vi "Scalar Bitpacked.vi"(8 "error in (no error)":errorcluster, 11 "Node Ptr":T1 format="%.0x") -> (0 "error out":errorcluster)   [LabVIEW 2018, in "FPGA Addon System Explorer.lvlib"]
uses:
  FPGA Addon System Explorer.lvlib
  <vilib>/NI VeriStand/Custom Device API/Custom Device API.lvlib
  Addon Shared/FPGA Addon Shared.lvlib
  Addon Shared/Types/FG Action.ctl
  Addon Shared/SubVIs/Constants.vi
  <vilib>/NI VeriStand/Custom Device API/Get Item Property (String).vi
  <vilib>/NI VeriStand/Custom Device API/Custom Device Item Ref.ctl
panel:
  out "Original Name":string
  in  "SHDocVw.IWebBrowser":refnum<k7>(container)
  in  "Reset":bool
  in  "Apply":bool
  in  "Number of Channels":u8
  in  "Header 2":cluster{"Section Name":string}={"Section Name"="Bitpacked Settings"}
  in  "Header":cluster{"Section Name":string}={"Section Name"="Section Settings"}
  in  "Description":string
  in  "Name":string
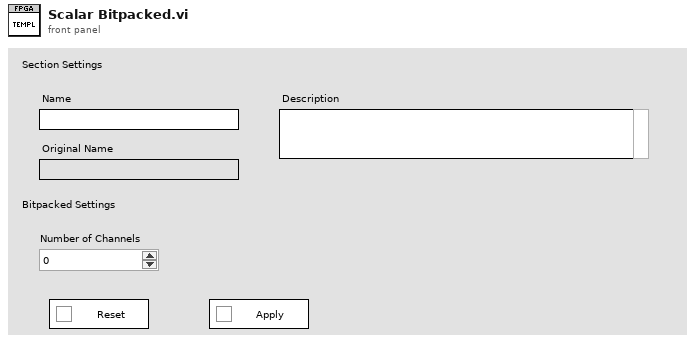
[diagram p1: front panel]
types:
  T1 = typedef "Custom Device API.lvlib/Custom Device Item Ref.ctl" = u64
  T2 = typedef "FPGA Addon Shared.lvlib/FG Action.ctl" = enum8{"GET", "SET"}
  T3 = typedef "FPGA Addon Shared.lvlib/Scalar Settings.ctl" = cluster{"Number of Channels":u8}
  T4 = typedef "FPGA Addon Shared.lvlib/Register Information.ctl" = cluster{"Name":string, "Data Type":T5, "Default Value":variant}
  T5 = typedef "FPGA Addon Shared.lvlib/Data Type.ctl" = enum8{"<Null>", "I8", "I16", "I32", "I64", "U8", "U16", "U32", "U64", "SGL", "Boolean", "Analog PWM In Settings", "Analog PWM In", "Digital PWM In Settings", "Digital PWM In", "Digital PWM Out", "Sine Out", "FXP+/-24.5", "FXP+/-16.5", "FXP+/-32.8", "FXP+/-64.32", "FXP+/-16.7", "FXP+/-20.5", "FXP+/-27.5", "FXP+/-32.16", "FXP+16.3", "FXP+18.3", "Digital Static In", "Digital Static Out", "Digital Static In Settings", "Digital WSS Out", "Quad Encoder Settings", "Quad Encoder In", "Group"}
  T6 = typedef "Custom Device API.lvlib/Custom Device Item Info.ctl" = cluster{"Name":string, "Is Channel":bool, "GUID":string, "Is Waveform":bool}
  T7 = typedef "Custom Device API.lvlib/Custom Device Commands.ctl" = enum16{"Default", "Item renamed", "Shutdown", "Dynamic button pressed"}
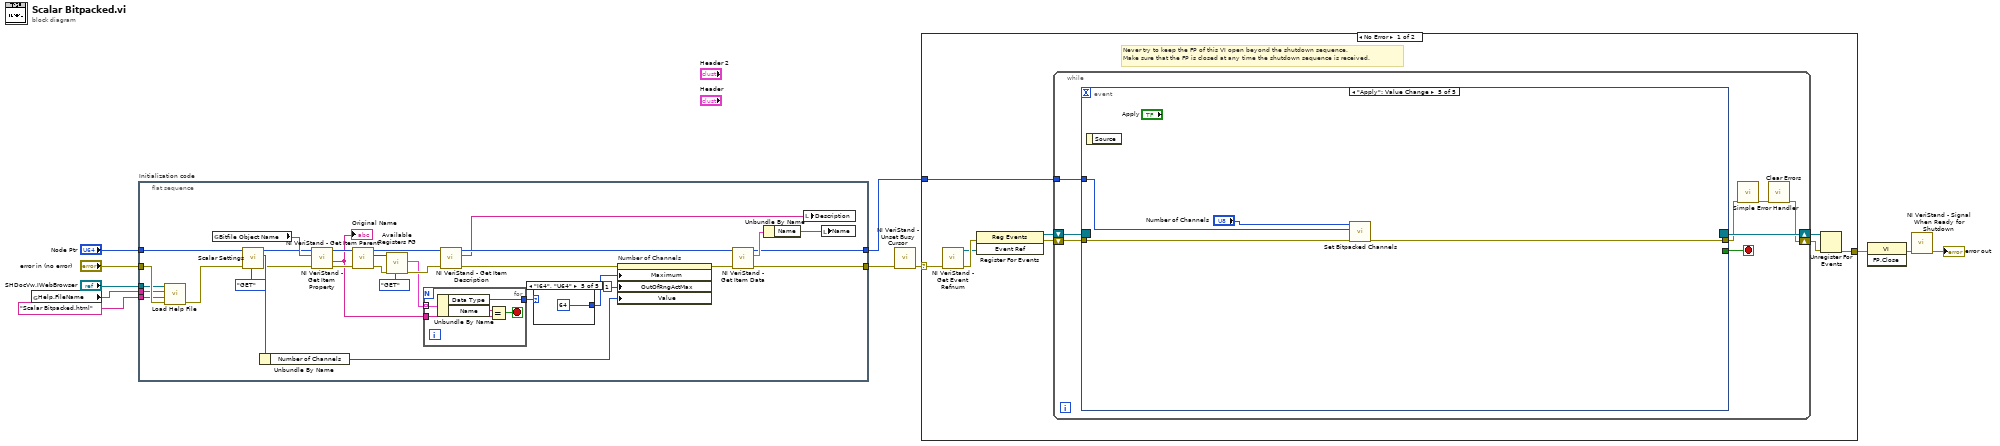
[diagram p0: block diagram]
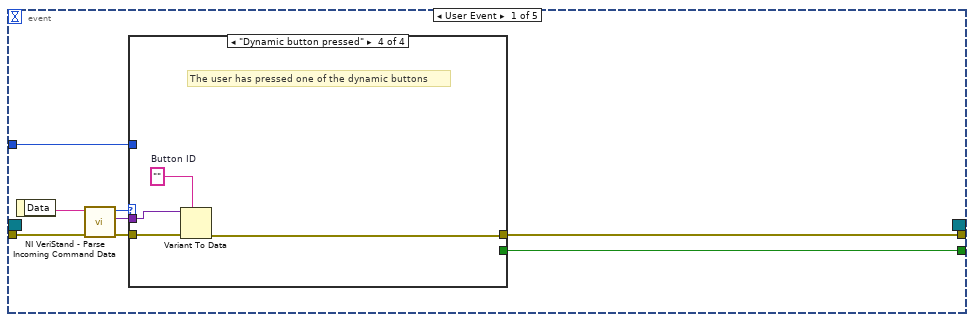
[diagram p2: hidden frame]
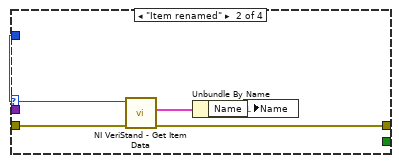
[diagram p4: hidden frame]
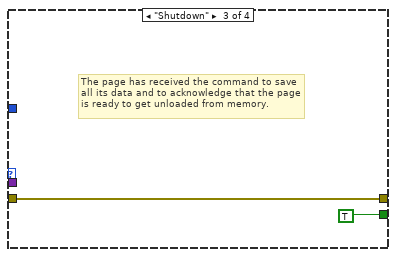
[diagram p5: hidden frame]
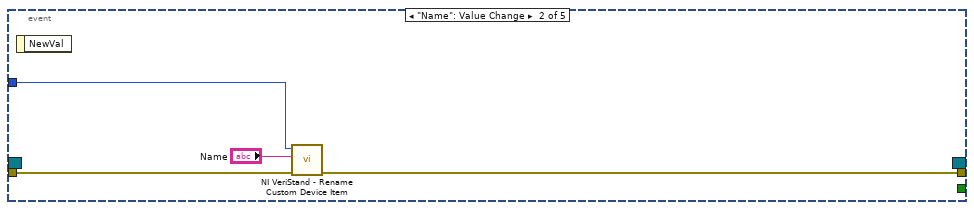
[diagram p6: hidden frame]
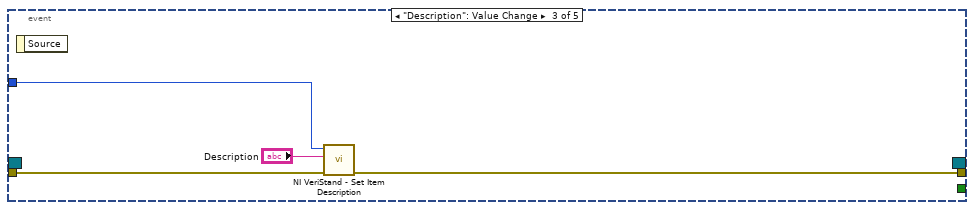
[diagram p7: hidden frame]
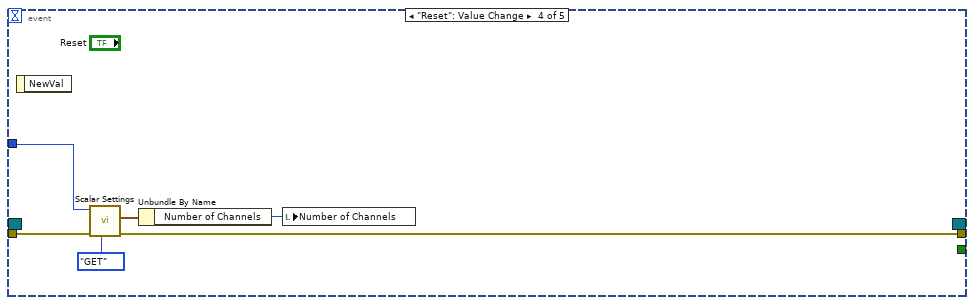
[diagram p8: hidden frame]
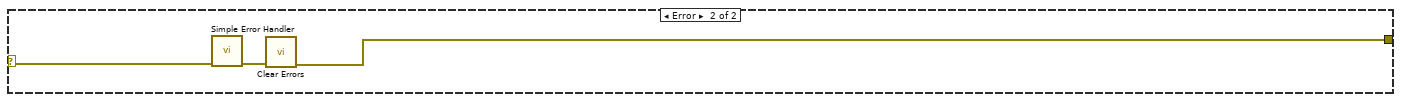
[diagram p9: hidden frame]
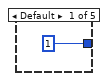
[diagram p10: hidden frame]
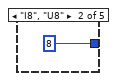
[diagram p11: hidden frame]
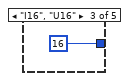
[diagram p12: hidden frame]
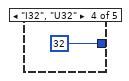
[diagram p13: hidden frame]
diagram:
  n1 = global read "Constants.vi" "Help.FileName"() -> (w1:string)
  n2 = flat-sequence "Initialization code" {
    tunnel: "error in (no error)" -> [w17]
    tunnel: "Node Ptr" -> [w25]
    tunnel: [w39] -> w8
    tunnel: [w40] -> w6
    tunnel: "SHDocVw.IWebBrowser" -> [w15]
    tunnel: w1 -> [w14]
    tunnel: "Scalar Bitpacked.html" ("HTML File") -> [w13]
    frame #0 {
      n3 = call "Load Help File.vi"("error in (no error)"=w17, "HTML File"=w13, "Main CHM File"=w14, "SHDocVw.IWebBrowser2"=w15) -> ("error out"=w16:errorcluster)  [unwired: 7 in]
      n4 = global read "Constants.vi" "Bitfile Object Name"() -> (w30:string)
      n5 = call "Scalar Settings.vi"("Action"=FG_Action."GET", "error in (no error)"=w16, "Item Ref"=w25) -> ("error out"=w24:errorcluster, "Scalar Settings"=w37:T3, "Item Ref out"=w23:T1)  [unwired: 6 in]
      n6 = Unbundle By Name(w37) -> ("Number of Channels"=w28:u8)
      n7 = call-poly <vilib>:"NI VeriStand - Get Item Property.vi"("error in (no error)"=w24, "Property Name"=w30, "Item Ref in"=w23) -> ("error out"=w21:errorcluster, "Value"=w12:string, "Item Ref out"=w22:T1)  [unwired: 5 in, 1 out]
      "Original Name" <- w12
      n8 = call <vilib>:"NI VeriStand - Get Item Parent.vi"("error in (no error)"=w21, "Item Ref in"=w22) -> ("error out"=w34:errorcluster, "Parent Ref"=w35:T1, "Item Ref out"=w36:T1)  [unwired: 6 in, 1 out]
      n9 = call "Available Registers FG.vi"("Action"=FG_Action."GET", "error in (no error)"=w34, "Item Ref"=w35) -> ("error out"=w33:errorcluster, "Available Registers"=w31:T4[])  [unwired: 6 in, 1 out]
      n10 = for {
        tunnel: w31 -> [w53] mode=indexing
        tunnel: w12 -> [w51]
        tunnel: [w49] -> w27
        stop <- w50 stop-if-true
        n11 = Unbundle By Name(w53) -> ("Data Type"=w49:T5, "Name"=w52:string)
        n12 = Equal?(x=w52, y=w51) -> (x = y?=w50:bool)
      }
      n13 = call <vilib>:"NI VeriStand - Get Item Description.vi"("error in (no error)"=w33, "Item Ref in"=w36) -> ("error out"=w20:errorcluster, "Description"=w42:string, "Item Ref out"=w43:T1)  [unwired: 7 out]
      n14 = case shown="\"I64\", \"U64\"" w27 {
        tunnel: [1 8 16 32 64] -> w26
        frame Default {
        }
        frame "I8", "U8" {
        }
        frame "I16", "U16" {
        }
        frame "I32", "U32" {
        }
        frame "I64", "U64" {
        }
      }
      n15 = property on="Number of Channels" class="DigNum (strict)"(error in=w20, "Maximum"=w26, "OutOfRngActMax"=u8 1 ("Response to Value Outside Limits:Maximum"), "Value"=w28) -> (error out=w19:errorcluster)  [unwired: 1 in, 1 out]
      n16 = call <vilib>:"NI VeriStand - Get Item Data.vi"("error in (no error)"=w19, "Item Ref in"=w43) -> ("error out"=w39:errorcluster, "Item Info"=w41:T6, "Item Ref out"=w40:T1)  [unwired: 7 out]
      n17 = Unbundle By Name(w41) -> ("Name"=w18:string)
      n18 = local write "Description"(w42) -> ()
      n19 = local write "Name"(w18) -> ()
    }
  }
  n20 = call <vilib>:"NI VeriStand - Unset Busy Cursor.vi"("error in (no error)"=w8) -> ("error out"=w7:errorcluster)  [unwired: 10 out]
  n21 = case shown="No Error" w7 {
    selector: w7 -> [w54 w111]
    tunnel: [w59 w109] -> w11
    tunnel: w6 -> [w55 _]
    frame No Error {
      # "Never try to keep the FP of this VI open beyond the shutdown sequence.\nMake sure that the FP is closed at any time the shutdown sequence is received."
      n22 = call <vilib>:"NI VeriStand - Get Event Refnum.vi"("error in (no error)"=w54) -> ("error out"=w62:errorcluster, "Event Ref"=w58:refnum<user-event>)  [unwired: 9 out]
      n23 = register-events(error in=w62, w58) -> (reference out=w56:refnum<event-registration>, error out=w57:errorcluster)  [unwired: 1 in]
      n24 = while {
        tunnel: w55 -> [w66]
        shift-right: [w63] -> w60
        shift-left: w57 -> [w69]
        shift-right: [w70] -> w61
        shift-left: w56 -> [w68]
        stop <- w67 stop-if-true
        n25 = event shown="[4] \"Apply\": Value Change" {
          selector: w68 -> [_ _ _ _ _]
          dyn-events: [_ _ _ _ _] -> w70
          timeout: _ -> [_ _ _ _ _]
          tunnel: w69 -> [w78 w94 w97 w104 w106]
          tunnel: [w74 _ _ _ _] -> w67
          tunnel: [w73 w93 w96 w100 w105] -> w65
          tunnel: w66 -> [w72 w92 w98 w102 w107]
          event User Event {
            n26 = event-data() -> ("Data"=w77:string)  [unwired: 1 out]
            n27 = call <vilib>:"NI VeriStand - Parse Incoming Command Data.vi"("error in (no error)"=w78, "Incoming data"=w77) -> ("error out"=w76:errorcluster, "Outgoing data"=w71:variant, "Action"=w75:T7)  [unwired: 7 out]
            n28 = case shown="\"Dynamic button pressed\"" w75 {
              tunnel: w76 -> [w79 w84 w85 w90]
              tunnel: [_ _ TRUE _] -> w74
              tunnel: [w79 w81 w85 w87] -> w73
              tunnel: w72 -> [_ w83 _ _]
              tunnel: w71 -> [_ _ _ w89]
              frame "Default", Default {
              }
              frame "Item renamed" {
                n29 = call <vilib>:"NI VeriStand - Get Item Data.vi"("error in (no error)"=w84, "Item Ref in"=w83) -> ("error out"=w81:errorcluster, "Item Info"=w82:T6)  [unwired: 8 out]
                n30 = Unbundle By Name(w82) -> ("Name"=w80:string)
                n31 = local write "Name"(w80) -> ()
              }
              frame "Shutdown" {
                # "The page has received the command to save all its data and to acknowledge that the page is ready to get unloaded from memory."
              }
              frame "Dynamic button pressed" {
                w88 = ""  # Button ID
                # "The user has pressed one of the dynamic buttons"
                n32 = Variant To Data(error in=w90, type=w88, Variant=w89) -> (error out=w87:errorcluster)  [unwired: 1 out]
              }
            }
          }
          event "Name": Value Change {
            n33 = event-data() -> ()  [unwired: 2 out]
            n34 = call <vilib>:"NI VeriStand - Rename Custom Device Item.vi"("error in (no error)"=w94, "New Name"="Name", "Item Ref in"=w92) -> ("error out"=w93:errorcluster)  [unwired: 1 in, 7 out]
          }
          event "Description": Value Change {
            n35 = event-data() -> ()  [unwired: 2 out]
            n36 = call <vilib>:"NI VeriStand - Set Item Description.vi"("error in (no error)"=w97, "Description"="Description", "Item Ref in"=w98) -> ("error out"=w96:errorcluster)  [unwired: 8 out]
          }
          event "Reset": Value Change {
            n37 = event-data() -> ()  [unwired: 2 out]
            n38 = call "Scalar Settings.vi"("Action"=FG_Action."GET", "error in (no error)"=w104, "Item Ref"=w102) -> ("error out"=w100:errorcluster, "Scalar Settings"=w101:T3)  [unwired: 6 in, 1 out]
            n39 = Unbundle By Name(w101) -> ("Number of Channels"=w99:u8)
            n40 = local write "Number of Channels"(w99) -> ()
          }
          event "Apply": Value Change {
            n41 = event-data() -> ()  [unwired: 2 out]
            n42 = call "Set Bitpacked Channels.vi"("error in (no error)"=w106, "Item Ref in"=w107, "Number of Channels"="Number of Channels") -> ("error out"=w105:errorcluster)  [unwired: 8 in]
          }
        }
        n43 = call <vilib>:"Simple Error Handler.vi"("error in (no error)"=w65) -> ("error out"=w64:errorcluster)  [unwired: 1 in, 7 out]
        n44 = call <vilib>:"Clear Errors.vi"("error in (no error)"=w64) -> ("error out"=w63:errorcluster)  [unwired: 1 in, 5 out]
      }
      n45 = Unregister For Events(event registration refnum=w61, error in=w60) -> (error out=w59:errorcluster)
    }
    frame Error {
      n46 = call <vilib>:"Simple Error Handler.vi"("error in (no error)"=w111) -> ("error out"=w110:errorcluster)  [unwired: 1 in, 7 out]
      n47 = call <vilib>:"Clear Errors.vi"("error in (no error)"=w110) -> ("error out"=w109:errorcluster)  [unwired: 1 in, 5 out]
    }
  }
  n48 = invoke class="VI" method="FP.Close"(error in=w11) -> (error out=w10:errorcluster)  [unwired: 2 in, 2 out]
  n49 = call <vilib>:"NI VeriStand - Signal When Ready for Shutdown.vi"("error in (no error)"=w10) -> ("error out"=→"error out":errorcluster)  [unwired: 10 out]
